vi "myRIO_BRig_FPGA_stateSelection.vi"(0 "I_selectionState":bool, 2 "I_selectRight":bool, 3 "I_selectWrong":bool, 5 "I_Left(F)_or_Right(T)":bool, 6 "I_ignoreWrong":bool, 8 "I_lickL":bool, 9 "I_laserEvent_Reward":bool, 10 "I_lickR":bool, 11 "I_laser_Reward":bool, 12 "I_lickObserved":bool, 13 "I_laserEvent_Wrong":bool, 15 "I_laser_Wrong":bool) -> (14 "output_I_lickObserved":bool, 22 "output__I_selectRight":bool, 23 "output__I_selectWrong":bool, 25 "output_I_startLaserEvent":bool, 26 "output_I_startLaser":bool)   [LabVIEW 2014]
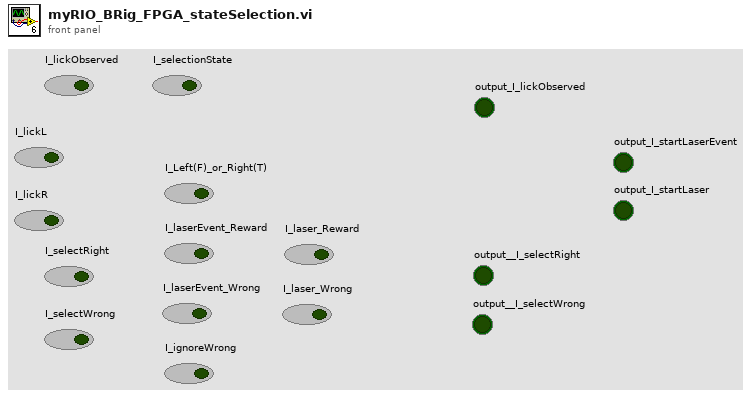
[diagram p1: front panel]
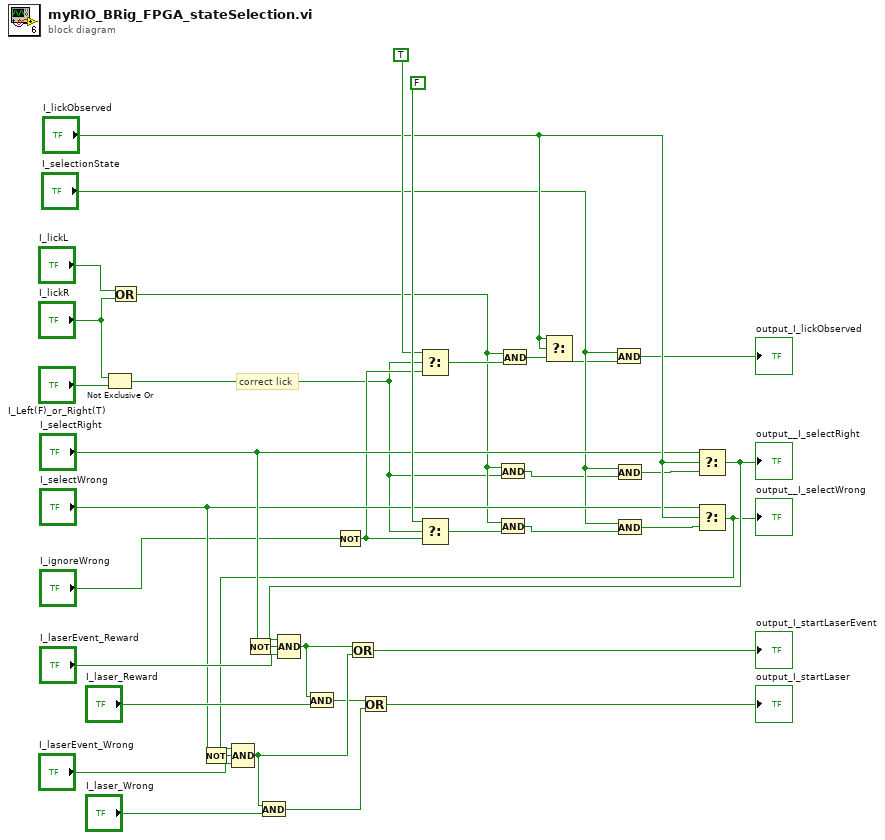
[diagram p0: block diagram]
diagram:
  # "correct lick"
  n1 = Not Exclusive Or(1:"I_Left(F)_or_Right(T)", 2:"I_lickR") -> (0:w1:bool)
  n2 = Or(x="I_lickL", y="I_lickR") -> (x .or. y?=w3:bool)
  n3 = Not(x="I_selectWrong") -> (.not. x?=w25:bool)
  n4 = Not(x="I_selectRight") -> (.not. x?=w27:bool)
  n5 = Not(x="I_ignoreWrong") -> (.not. x?=w19:bool)
  n6 = Select(t=TRUE, s=w1, f=w19) -> (s? t:f=w7:bool)
  n7 = Select(t=FALSE ("f"), s=w1, f=w19) -> (s? t:f=w4:bool)
  n8 = And(x=w3, y=w1) -> (x .and. y?=w5:bool)
  n9 = And(x=w3, y=w4) -> (x .and. y?=w2:bool)
  n10 = And(x=w3, y=w7) -> (x .and. y?=w6:bool)
  n11 = Select(t="I_lickObserved", s="I_lickObserved", f=w6) -> (s? t:f=w9:bool)
  n12 = And(x="I_selectionState", y=w9) -> (x .and. y?=→"output_I_lickObserved":bool)
  n13 = And(x="I_selectionState", y=w5) -> (x .and. y?=w11:bool)
  n14 = And(x="I_selectionState", y=w2) -> (x .and. y?=w12:bool)
  n15 = Select(t="I_selectRight", s="I_lickObserved", f=w11) -> (s? t:f=w28:bool)
  "output__I_selectRight" <- w28
  n16 = Compound Arithmetic op=AND(w28, w27, "I_laserEvent_Reward") -> (w18:bool)
  n17 = And(x=w18, y="I_laser_Reward") -> (x .and. y?=w16:bool)
  n18 = Select(t="I_selectWrong", s="I_lickObserved", f=w12) -> (s? t:f=w22:bool)
  "output__I_selectWrong" <- w22
  n19 = Compound Arithmetic op=AND(w22, w25, "I_laserEvent_Wrong") -> (w17:bool)
  n20 = And(x=w17, y="I_laser_Wrong") -> (x .and. y?=w15:bool)
  n21 = Or(x=w18, y=w17) -> (x .or. y?=→"output_I_startLaserEvent":bool)
  n22 = Or(x=w16, y=w15) -> (x .or. y?=→"output_I_startLaser":bool)
